vi "1C.1 Camera - PixelToUTM.vi"(8 "Resolution of camera in pixels":dbl=1384.0, 9 "Width of camera view in meters":dbl=4.648, 10 "Found Marker Position in (pixels)":cluster{"Y":dbl, "X":i32}) -> (2 "UTM Location Out":T1)   [LabVIEW 2011]
doc: "Converts the location determined from the camera image to \"UTM Coordinates\", where the reference point is the bottom left of the image. Takes in the pixel coordinates of the boat, returns UTM Coordinates. Can also optionally take in the camera resolution and the width of view."
uses:
  2-RIO/2 Typedefs/UTM Location.ctl
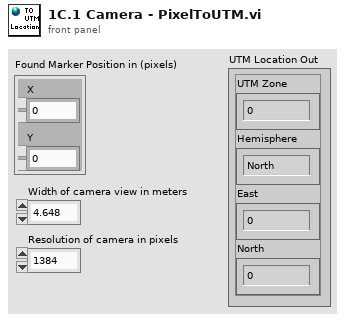
[diagram p1: front panel]
types:
  T1 = typedef "UTM Location.ctl" = cluster{"UTM Zone":dbl, "Hemisphere":enum16{"North", "South"}, "East":dbl, "North":dbl}
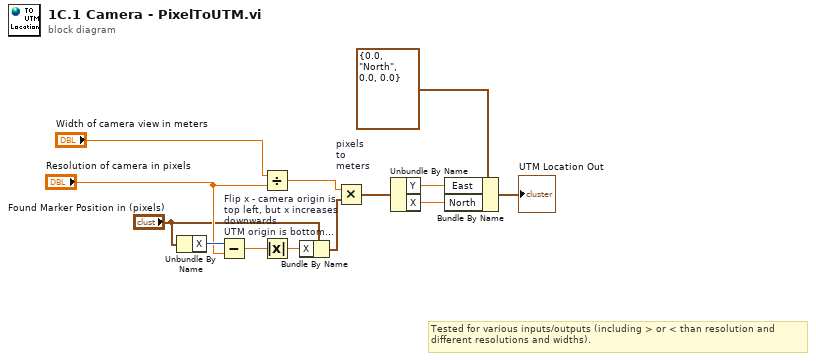
[diagram p0: block diagram]
diagram:
  # "Tested for various inputs/outputs (including > or < than resolution and\ndifferent resolutions and widths)."
  n1 = Unbundle By Name("Found Marker Position in (pixels)") -> ("X"=w13:i32)
  n2 = Subtract "Flip x - camera origin is top left, but x increases downwards.\nUTM origin is bottom left."(x=w13, y="Resolution of camera in pixels") -> (x-y=w12:dbl)
  n3 = Divide(x="Width of camera view in meters", y="Resolution of camera in pixels") -> (x/y=w2:dbl)
  n4 = Absolute Value(x=w12) -> (abs(x)=w11:dbl)
  n5 = Bundle By Name(cluster="Found Marker Position in (pixels)", "X"=w11) -> (w4:cluster{"Y":dbl, "X":i32})
  n6 = Multiply "pixels\nto\nmeters"(x=w2, y=w4) -> (x*y=w10:cluster{"Y":dbl, "X":dbl})
  n7 = Unbundle By Name(w10) -> ("Y"=w8:dbl, "X"=w1:dbl)
  n8 = Bundle By Name(cluster=T1 {"UTM Zone"=0.0, "Hemisphere"=enum."North", "East"=0.0, "North"=0.0} ("UTM Location"), "East"=w8, "North"=w1) -> (→"UTM Location Out":T1)
